vi "superhetero.vi"() -> ()   [LabVIEW 2009]
uses:
  <vilib>/Analysis/NI_AALBase.lvlib
panel:
  in  "数値 2":dbl
  in  "数値":dbl
  out "歪み率":dbl
  out "出力":cluster{dbl[], dbl[]}(graph) caption="XYグラフ"
  out "送信波":cluster{dbl[], dbl[]}(graph)
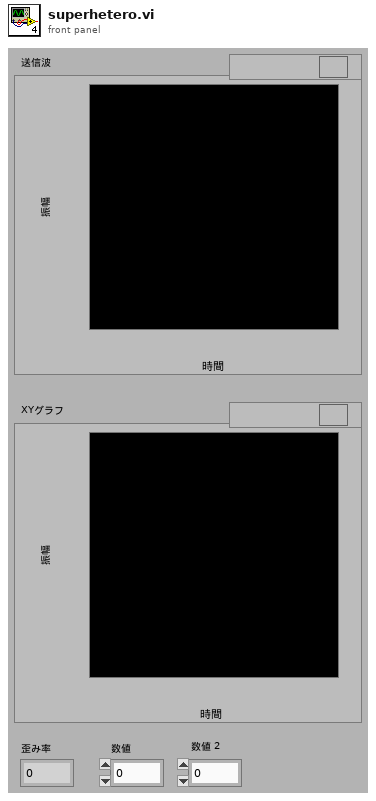
[diagram p1: front panel]
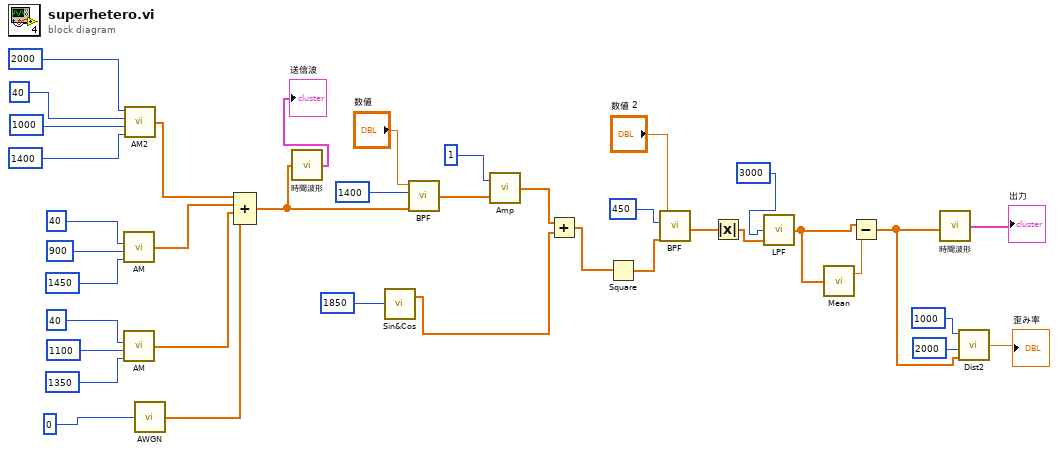
[diagram p0: block diagram]
diagram:
  n1 = call "AM.vi"("変調度 [%]"=40, "変調周波数 [Hz]"=900, "搬送波周波数 [kHz]"=1450) -> ("変調波"=w32:dbl[])  [unwired: 2 in]
  n2 = call "AM.vi"("変調度 [%]"=40, "変調周波数 [Hz]"=1100, "搬送波周波数 [kHz]"=1350) -> ("変調波"=w31:dbl[])  [unwired: 2 in]
  n3 = call "AM2.vi"("搬送波周波数 [kHz]"=1400, "変調周波数1 [Hz]"=1000, "変調度 [%]"=40, "変調周波数2 [Hz]"=2000) -> ("変調波"=w5:dbl[])  [unwired: 2 in]
  n4 = call "AWGN.vi"("振幅値"=0) -> ("出力"=w30:dbl[])
  n5 = Compound Arithmetic op=ADD(w5, w32, w31, w30) -> (w27:dbl[])
  n6 = call "時間波形.vi"("入力"=w27) -> ("時間波形"=→"送信波":cluster{dbl[], dbl[]})
  n7 = call "Sin&Cos.vi"("周波数[kHz]"=1850) -> ("sin"=w14:dbl[])  [unwired: 1 out]
  n8 = call "BPF.vi"("X"=w27, "中心周波数 [kHz]"=1400, "Q"="数値") -> ("BPF出力"=w16:dbl[])  [unwired: 1 in]
  n9 = call "Amp.vi"("入力"=w16, "増幅率"=1) -> ("出力"=w15:dbl[])
  n10 = Add(x=w15, y=w14) -> (x+y=w13:dbl[])
  n11 = Square(x=w13) -> (x^2=w12:dbl[])
  n12 = call "BPF.vi"("X"=w12, "中心周波数 [kHz]"=450, "Q"="数値 2") -> ("BPF出力"=w20:dbl[])  [unwired: 1 in]
  n13 = Absolute Value(x=w20) -> (abs(x)=w19:dbl[])
  n14 = call "LPF.vi"("入力"=w19, "カットオフ周波数 [Hz]"=3000) -> ("LPF出力"=w17:dbl[])  [unwired: 1 in]
  n15 = call <vilib>:"Mean.vi"("X"=w17) -> ("mean"=w18:dbl)  [unwired: 1 out]
  n16 = Subtract(x=w17, y=w18) -> (x-y=w2:dbl[])
  n17 = call "時間波形.vi"("入力"=w2) -> ("時間波形"=→"出力":cluster{dbl[], dbl[]})
  n18 = call "Dist2.vi"("入力"=w2, "基本周波数1 [Hz]"=2000, "基本周波数2 [Hz]"=1000) -> ("ひずみ率"=→"歪み率":dbl)  [unwired: 1 in]
